vi "Gather Statistics.vi"(10 "JSON Scalar":refnum<class "JSON Scalar.lvclass">, 11 "JSON Value In":refnum<class "JSON Value.lvclass">) -> (3 "JSON Statistic or Object":refnum<class "JSON Value.lvclass">)   [LabVIEW 2020, in "Library Commun.lvlib" / "JSON Scalar.lvclass"]
uses:
  JSON Scalar.lvclass
  JSON Value/JSON Value.lvclass
  C:/Users/ngarcin/OneDrive - Altyor/Standard TB/Class/JSON API/JSON Value/JSON Value.lvclass
  Statistics/JSON Statistics.lvclass
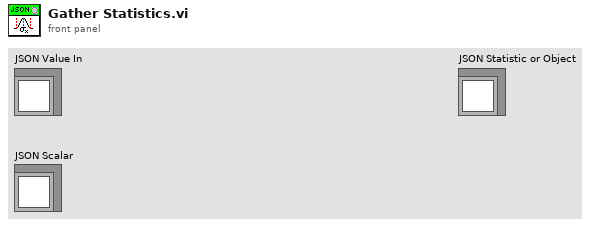
[diagram p1: front panel]
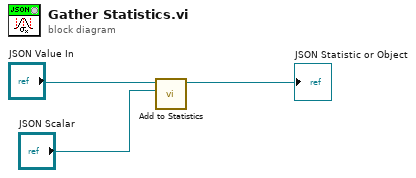
[diagram p0: block diagram]
diagram:
  n1 = call-dynamic "Add to Statistics.vi"("Non Object"="JSON Scalar", "JSON Value In"="JSON Value In") -> ("JSON Statistics out"=→"JSON Statistic or Object":refnum<class "JSON Statistics.lvclass">)  [unwired: 9 in]
